vi "convert measurement file to html table.vi"(2 "target file (new html document)":path, 3 "source  file (spreadsheet file)":path) -> (1 "target file path (copy)":path)   [LabVIEW 2009]
uses:
  <vilib>/Utility/file.llb/Read From Spreadsheet File (string).vi
panel:
  out "column #":i32
  out "row #":i32
  out "progress (row)":i32(slide) scale=0.0..838.0
  out "progress (column)":i32(slide) scale=0.0..3.0
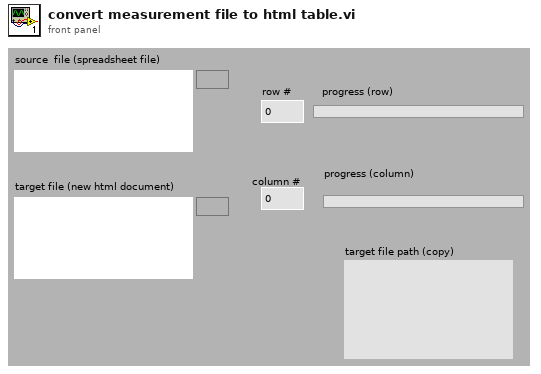
[diagram p1: front panel]
types:
  T1 = enum16{"open", "replace", "create", "open or create", "replace or create", "replace or create with confirmation"}
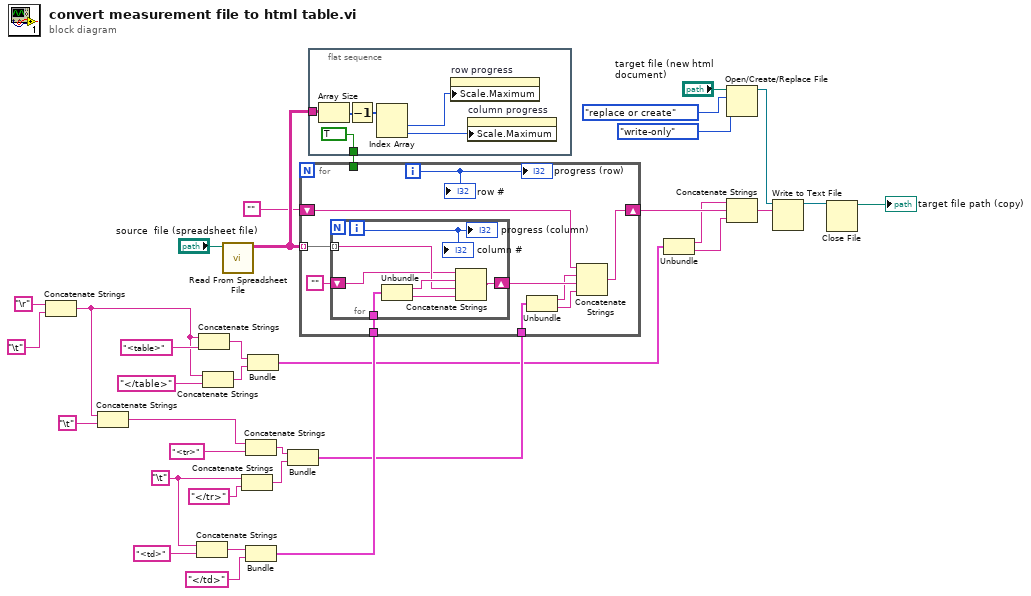
[diagram p0: block diagram]
diagram:
  w2 = "\t"
  n1 = Concatenate Strings("\r", "\t") -> (w28:string)
  n2 = Concatenate Strings(w28, "\t") -> (w24:string)
  n3 = Concatenate Strings(w2, "<td>") -> (w5:string)
  n4 = Concatenate Strings(w28, "<table>") -> (w32:string)
  n5 = Concatenate Strings(w28, "</table>") -> (w31:string)
  n6 = call-poly <vilib>:"Read From Spreadsheet File.vi"("file path (dialog if empty)"="source  file (spreadsheet file)") -> ("all rows"=w12:string[][])  [unwired: 6 in, 4 out]
  n7 = Concatenate Strings(w2, "</tr>") -> (w1:string)
  n8 = Concatenate Strings(w24, "<tr>") -> (w25:string)
  n9 = Bundle(w5, "</td>") -> (w23:cluster{string, string})  [unwired: 1 in]
  n10 = Bundle(w32, w31) -> (w21:cluster{string, string})  [unwired: 1 in]
  n11 = Bundle(w25, w1) -> (w22:cluster{string, string})  [unwired: 1 in]
  n12 = for {
    tunnel: w12 -> [w44] mode=indexing
    tunnel: w23 -> [w43]
    tunnel: w22 -> [w42]
    shift-right: [w37] -> w20
    shift-left: "" -> [w38]
    tunnel: w11 -> [_]
    i -> [w36]
    n13 = for {
      tunnel: w44 -> [w48] mode=indexing
      tunnel: w43 -> [w51]
      shift-right: [w47] -> w41
      shift-left: "" -> [w46]
      i -> [w45]
      n14 = Unbundle(w51) -> (w49:string, w50:string)
      n15 = Concatenate Strings(w46, w49, w48, w50) -> (w47:string)
      "progress (column)" <- w45
      "column #" <- w45
    }
    n16 = Unbundle(w42) -> (w39:string, w40:string)
    n17 = Concatenate Strings(w38, w39, w41, w40) -> (w37:string)
    "progress (row)" <- w36
    "row #" <- w36
  }
  n18 = flat-sequence {
    tunnel: w12 -> [w57]
    tunnel: [TRUE] -> w11
    frame #0 {
      n19 = Array Size(array=w57) -> (size(s)=w56:i32[])
      n20 = Decrement(x=w56) -> (x-1=w55:i32[])
      n21 = Index Array(array=w55) -> (element #1=w54:i32, element #2=w53:i32)  [unwired: 2 in]
      n22 = property on="row progress" class="Slide (strict)"("Scale.Maximum"=w54) -> ()  [unwired: 2 in, 2 out]
      n23 = property on="column progress" class="Slide (strict)"("Scale.Maximum"=w53) -> ()  [unwired: 2 in, 2 out]
    }
  }
  n24 = Unbundle(w21) -> (w18:string, w19:string)
  n25 = Open/Create/Replace File(file path (use dialog)="target file (new html document)", operation (0:open)=T1."replace or create", access (0:read/write)=enum16{"read/write", "read-only", "write-only"}."write-only") -> (refnum out=w17:refnum<file>)  [unwired: 3 in, 2 out]
  n26 = Concatenate Strings(w18, w20, w19) -> (w16:string)
  n27 = Write to Text File(file (use dialog)=w17, text=w16) -> (refnum out=w15:refnum<file>)  [unwired: 2 in, 2 out]
  n28 = Close File(refnum=w15) -> (path=→"target file path (copy)":path)  [unwired: 1 in, 1 out]
